vi "SFOAE-Update Stimulus.vi"(0 "AO Runtime in":T1, 11 "error in (no error)":errorcluster) -> (4 "AO Runtime out":T1, 15 "error out":errorcluster)   [LabVIEW 2020]
uses:
  Typedefs/SFOAE-AO Runtime Data.ctl
  epl-vi-lib/Utility VIs/Math VIs/LinSpace (x0-dx-npts).vi
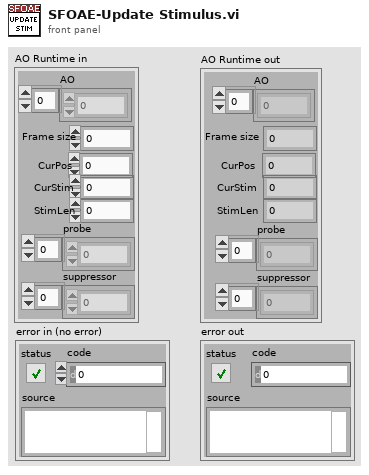
[diagram p1: front panel]
types:
  T1 = typedef "SFOAE-AO Runtime Data.ctl" = cluster{"AO":i32[], "Frame size":i32, "CurPos":i32, "probe":dbl[], "suppressor":dbl[], "CurStim":i32, "StimLen":i32}
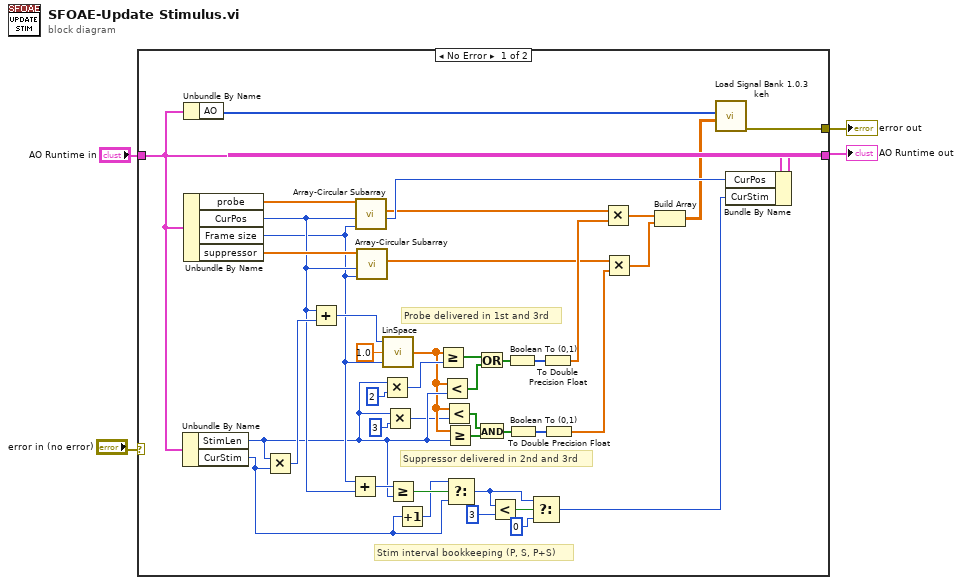
[diagram p0: block diagram]
diagram:
  n1 = case shown="No Error" "error in (no error)" {
    selector: "error in (no error)" -> [_ w47]
    tunnel: "AO Runtime in" -> [w24 w48]
    tunnel: [w44 w48] -> w2
    tunnel: [w40 w47] -> w4
    frame No Error {
      # "Stim interval bookkeeping (P, S, P+S)"
      # "Suppressor delivered in 2nd and 3rd"
      # "Probe delivered in 1st and 3rd"
      n2 = Unbundle By Name(w24) -> ("StimLen"=w8:i32, "CurStim"=w19:i32)
      n3 = Unbundle By Name(w24) -> ("AO"=w41:i32[])
      n4 = Unbundle By Name(w24) -> ("probe"=w46:dbl[], "CurPos"=w12:i32, "Frame size"=w11:i32, "suppressor"=w45:dbl[])
      n5 = Multiply(x=w8, y=w19) -> (x*y=w22:i32)
      n6 = Add(x=w12, y=w22) -> (x+y=w23:i32)
      n7 = Add(x=w11, y=w12) -> (x+y=w21:i32)
      n8 = call "Array-Circular Subarray.vi"("Npts"=w11, "Offset (in)"=w12, "Array"=w46) -> ("Offset (out)"=w43:i32, "Subarray"=w32:dbl[])  [unwired: 7 in]
      n9 = call "Array-Circular Subarray.vi"("Npts"=w11, "Offset (in)"=w12, "Array"=w45) -> ("Subarray"=w27:dbl[])  [unwired: 7 in, 1 out]
      n10 = Multiply(x=w8, y=2) -> (x*y=w37:i32)
      n11 = call-poly "LinSpace.vi"("npts"=w11, "dx"=1.0, "x0"=w23) -> ("Array"=w7:dbl[])  [unwired: 1 in, 1 out]
      n12 = Multiply(x=w8, y=3) -> (x*y=w6:i32)
      n13 = Greater Or Equal?(x=w21, y=w8) -> (x >= y?=w20:bool)
      n14 = Increment(x=w19) -> (x+1=w18:i32)
      n15 = Greater Or Equal?(x=w7, y=w37) -> (x >= y?=w36:bool[])
      n16 = Less?(x=w7, y=w8) -> (x < y?=w35:bool[])
      n17 = Less?(x=w7, y=w6) -> (x < y?=w5:bool[])
      n18 = Greater Or Equal?(x=w7, y=w8) -> (x >= y?=w28:bool[])
      n19 = Select(t=w18, s=w20, f=w19) -> (s? t:f=w15:i32)
      n20 = Or(x=w36, y=w35) -> (x .or. y?=w34:bool[])
      n21 = And(x=w5, y=w28) -> (x .and. y?=w10:bool[])
      n22 = Less?(x=w15, y=3) -> (x < y?=w16:bool)
      n23 = Boolean To (0,1)(Boolean=w34) -> (0, 1=w33:i16[])
      n24 = Boolean To (0,1)(Boolean=w10) -> (0, 1=w29:i16[])
      n25 = Select(t=w15, s=w16, f=0) -> (s? t:f=w14:i32)
      n26 = To Double Precision Float(number=w33) -> (double precision float=w31:dbl[])
      n27 = To Double Precision Float(number=w29) -> (double precision float=w26:dbl[])
      n28 = Multiply(x=w32, y=w31) -> (x*y=w30:dbl[])
      n29 = Multiply(x=w27, y=w26) -> (x*y=w25:dbl[])
      n30 = Build Array(w30, w25) -> (w42:dbl[][])
      n31 = call "Load Signal Bank 1.0.3 keh.vi"("Input array"=w42, "Active AO Array"=w41) -> ("error out"=w40:errorcluster)  [unwired: 7 in, 2 out]
      n32 = Bundle By Name(cluster=w24, "CurPos"=w43, "CurStim"=w14) -> (w44:T1)
    }
    frame Error {
    }
  }
  "error out" <- w4
  "AO Runtime out" <- w2
